vi "toCompiledXml.vi"(8 "error in (no error)":errorcluster, 11 "RampEvent in":refnum<class "RampEvent.lvclass">) -> (0 "error out":errorcluster, 2 "compiledXML":refnum<class "xmlNode.lvclass">, 3 "RampEvent out":refnum<class "RampEvent.lvclass">)   [LabVIEW 2011, in "Tools.lvlib" / "Scripting.lvlib" / "RampEvent.lvclass"]
uses:
  RampEvent.lvclass
  xmlNode/xmlNode.lvclass
  DatabaseHelpers/Database Objects/Channel/Channel.lvclass
  ScriptEvent.lvclass
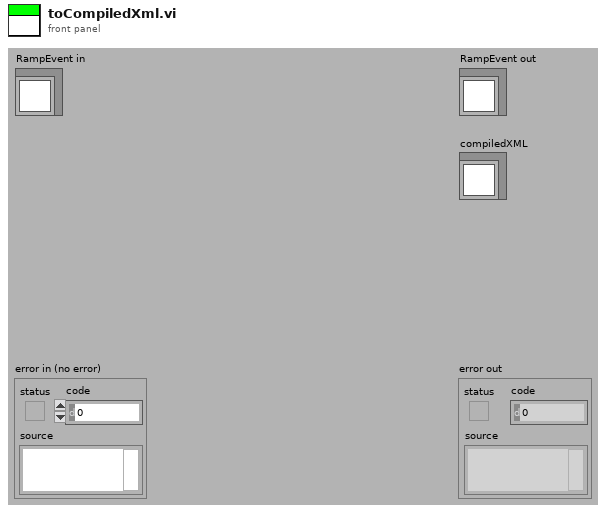
[diagram p1: front panel]
types:
  T1 = cluster{"attributeName":string, "channel_name":string}
  T2 = cluster{"attributeName":string, "channel_name":string}[]
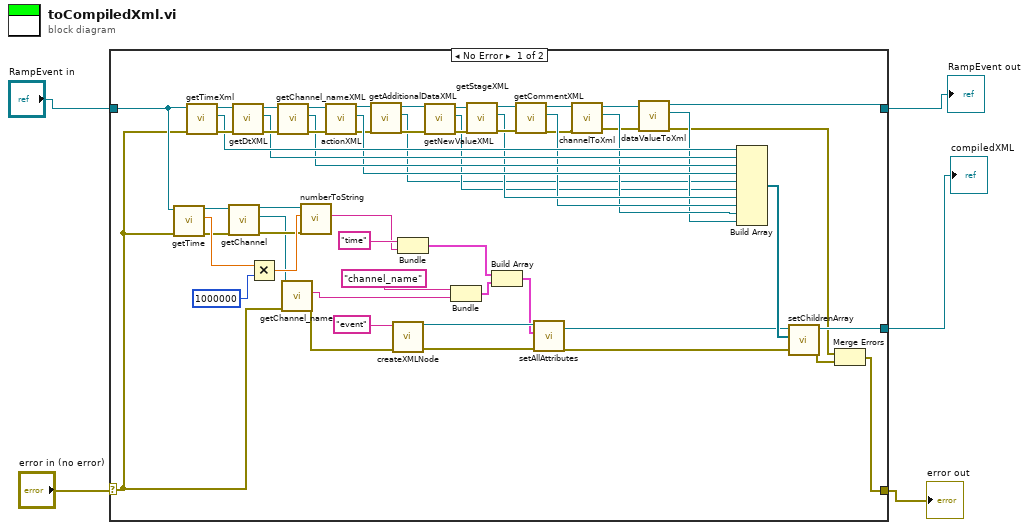
[diagram p0: block diagram]
diagram:
  n1 = case shown="No Error" "error in (no error)" {
    selector: "error in (no error)" -> [w11 w64]
    tunnel: [w41 w64] -> w1
    tunnel: [w21 w63] -> w4
    tunnel: "RampEvent in" -> [w13 w63]
    tunnel: [w43 _] -> w3
    frame No Error {
      n2 = call "getTime.vi"("error in (no error)"=w11, "ScriptEvent.lvclass in"=w13) -> ("error out"=w9:errorcluster, "time"=w12:dbl, "ScriptEvent.lvclass out"=w10:refnum<class "RampEvent.lvclass">)  [unwired: 7 in]
      n3 = call "getTimeXml.vi"("error in (no error)"=w11, "ScriptEvent in"=w13) -> ("error out"=w60:errorcluster, "timeXML"=w50:refnum<class "xmlNode.lvclass">, "ScriptEvent out"=w55:refnum<class "RampEvent.lvclass">)  [unwired: 7 in]
      n4 = call-dynamic "getChannel.vi"("error in (no error)"=w9, "ScriptEvent.lvclass in"=w10) -> ("error out"=w8:errorcluster, "Channel.lvclass"=w6:refnum<class "Channel.lvclass">, "ScriptEvent.lvclass out"=w7:refnum<class "RampEvent.lvclass">)  [unwired: 7 in]
      n5 = call "getDtXML.vi"("error in (no error)"=w60, "ScriptEvent in"=w55) -> ("error out"=w59:errorcluster, "dtXML"=w49:refnum<class "xmlNode.lvclass">, "ScriptEvent out"=w54:refnum<class "RampEvent.lvclass">)  [unwired: 7 in]
      n6 = Multiply(x=w12, y=1000000) -> (x*y=w29:dbl)
      n7 = call "getChannel_nameXML.vi"("error in (no error)"=w59, "ScriptEvent in"=w54) -> ("error out"=w58:errorcluster, "channel_nameXML"=w48:refnum<class "xmlNode.lvclass">, "ScriptEvent out"=w53:refnum<class "RampEvent.lvclass">)  [unwired: 7 in]
      n8 = call "getChannel_name.vi"("error in (no error)"=w11, "Channel.lvclass in"=w6) -> ("error out"=w61:errorcluster, "channel_name"=w38:string)  [unwired: 7 in, 1 out]
      n9 = call "numberToString.vi"("error in (no error)"=w8, "Numeric"=w29, "ScriptEvent in"=w7) -> ("String"=w28:string)  [unwired: 6 in, 2 out]
      n10 = call "actionXML.vi"("error in (no error)"=w58, "ScriptEvent in"=w53) -> ("error out"=w18:errorcluster, "actionXml"=w47:refnum<class "xmlNode.lvclass">, "ScriptEvent out"=w19:refnum<class "RampEvent.lvclass">)  [unwired: 7 in]
      n11 = call-dynamic "getAdditionalDataXML.vi"("error in (no error)"=w18, "RampEvent in"=w19) -> ("error out"=w17:errorcluster, "additionalDataXML"=w14:refnum<class "xmlNode.lvclass">, "RampEvent out"=w16:refnum<class "RampEvent.lvclass">)  [unwired: 7 in]
      n12 = call "createXMLNode.vi"("error in (no error)"=w61, "name"="event") -> ("error out"=w33:errorcluster, "xmlNode out"=w37:refnum<class "xmlNode.lvclass">)  [unwired: 8 in]
      n13 = Bundle("attributeName"="time", "String"=w28) -> (w36:cluster{"attributeName":string, "String":string})  [unwired: 1 in]
      n14 = call-dynamic "getNewValueXML.vi"("error in (no error)"=w17, "RampEvent in"=w16) -> ("error out"=w57:errorcluster, "newValueXML"=w15:refnum<class "xmlNode.lvclass">, "RampEvent out"=w52:refnum<class "RampEvent.lvclass">)  [unwired: 7 in]
      n15 = Bundle("attributeName"="channel_name", "channel_name"=w38) -> (w35:T1)  [unwired: 1 in]
      n16 = call "getStageXML.vi"("error in (no error)"=w57, "ScriptEvent in"=w52) -> ("error out"=w56:errorcluster, "stageXML"=w46:refnum<class "xmlNode.lvclass">, "ScriptEvent out"=w51:refnum<class "RampEvent.lvclass">)  [unwired: 7 in]
      n17 = Build Array(w36, w35) -> (w34:T2)
      n18 = call "getCommentXML.vi"("error in (no error)"=w56, "ScriptEvent in"=w51) -> ("error out"=w26:errorcluster, "commentXML"=w45:refnum<class "xmlNode.lvclass">, "ScriptEvent out"=w27:refnum<class "RampEvent.lvclass">)  [unwired: 7 in]
      n19 = call-dynamic "setAllAttributes.vi"("error in (no error)"=w33, "attributes"=w34, "xmlNode in"=w37) -> ("error out"=w32:errorcluster, "xmlNode out"=w31:refnum<class "xmlNode.lvclass">)  [unwired: 7 in]
      n20 = call "channelToXml.vi"("error in (no error)"=w26, "ScriptEvent in"=w27) -> ("error out"=w23:errorcluster, "xmlNode"=w25:refnum<class "xmlNode.lvclass">, "ScriptEvent out"=w24:refnum<class "RampEvent.lvclass">)  [unwired: 7 in]
      n21 = call-dynamic "dataValueToXml.vi"("error in (no error)"=w23, "RampEvent in"=w24) -> ("error out"=w20:errorcluster, "dataValueXml"=w22:refnum<class "xmlNode.lvclass">, "RampEvent out"=w21:refnum<class "RampEvent.lvclass">)  [unwired: 7 in]
      n22 = Build Array(w50, w49, w48, w47, w14, w15, w46, w45, w25, w22) -> (w44:refnum<class "xmlNode.lvclass">[])
      n23 = call-dynamic "setChildrenArray.vi"("error in (no error)"=w32, "Children"=w44, "xmlNode.lvclass in"=w31) -> ("error out"=w42:errorcluster, "xmlNode.lvclass out"=w43:refnum<class "xmlNode.lvclass">)  [unwired: 7 in]
      n24 = Merge Errors(w20, w42) -> (w41:errorcluster)
    }
    frame Error {
    }
  }
  "error out" <- w1
  "RampEvent out" <- w4
  "compiledXML" <- w3
